vi "Main.vi"() -> ()   [LabVIEW 2011]
uses:
  <vilib>/Utility/miscctls.llb/LVPointTypeDef.ctl
  typedefs/control_references_cluster.ctl
  typedefs/state_cluster.ctl
  typedefs/state_enum.ctl
  <vilib>/DAQmx/write.llb/DAQmx Write (Analog 1D DBL NChan 1Samp).vi
  <vilib>/DAQmx/write.llb/DAQmx Write (Analog 2D DBL NChan NSamp).vi
  subvis/global_image_size.vi
  <vilib>/DAQmx/create/channels.llb/DAQmx Create Channel (AO-Voltage-Basic).vi
  <vilib>/DAQmx/configure/timing.llb/DAQmx Timing (Sample Clock).vi
  <vilib>/DAQmx/miscellaneous.llb/DAQmx Fill In Error Info.vi
  Program Files/National Instruments/LabVIEW 2011/resource/objmgr/daqmx.rc
panel:
  out "SCORE":dbl(knob) scale=0.0..100.0 scale format="%#.0f"
  in  "Play":bool
  in  "Zeit pro Zelle":i32=1 min=1 max=10 step=1
  out "Internal quit":bool
  out "Pfadlänge":dbl format="%#.0f"
  out "Image":picture
  in  "Quit":bool
  out "Signal Qualität":i32(slide) scale=0.0..10.0
  out "Anzahl Neurone":u16(slide) scale=0.0..60.0
  out "Geschwindigkeit":dbl(slide) scale=0.01..1.0 scale format="%#.3g"
  # "Institut für Hirnforschung, UZH"
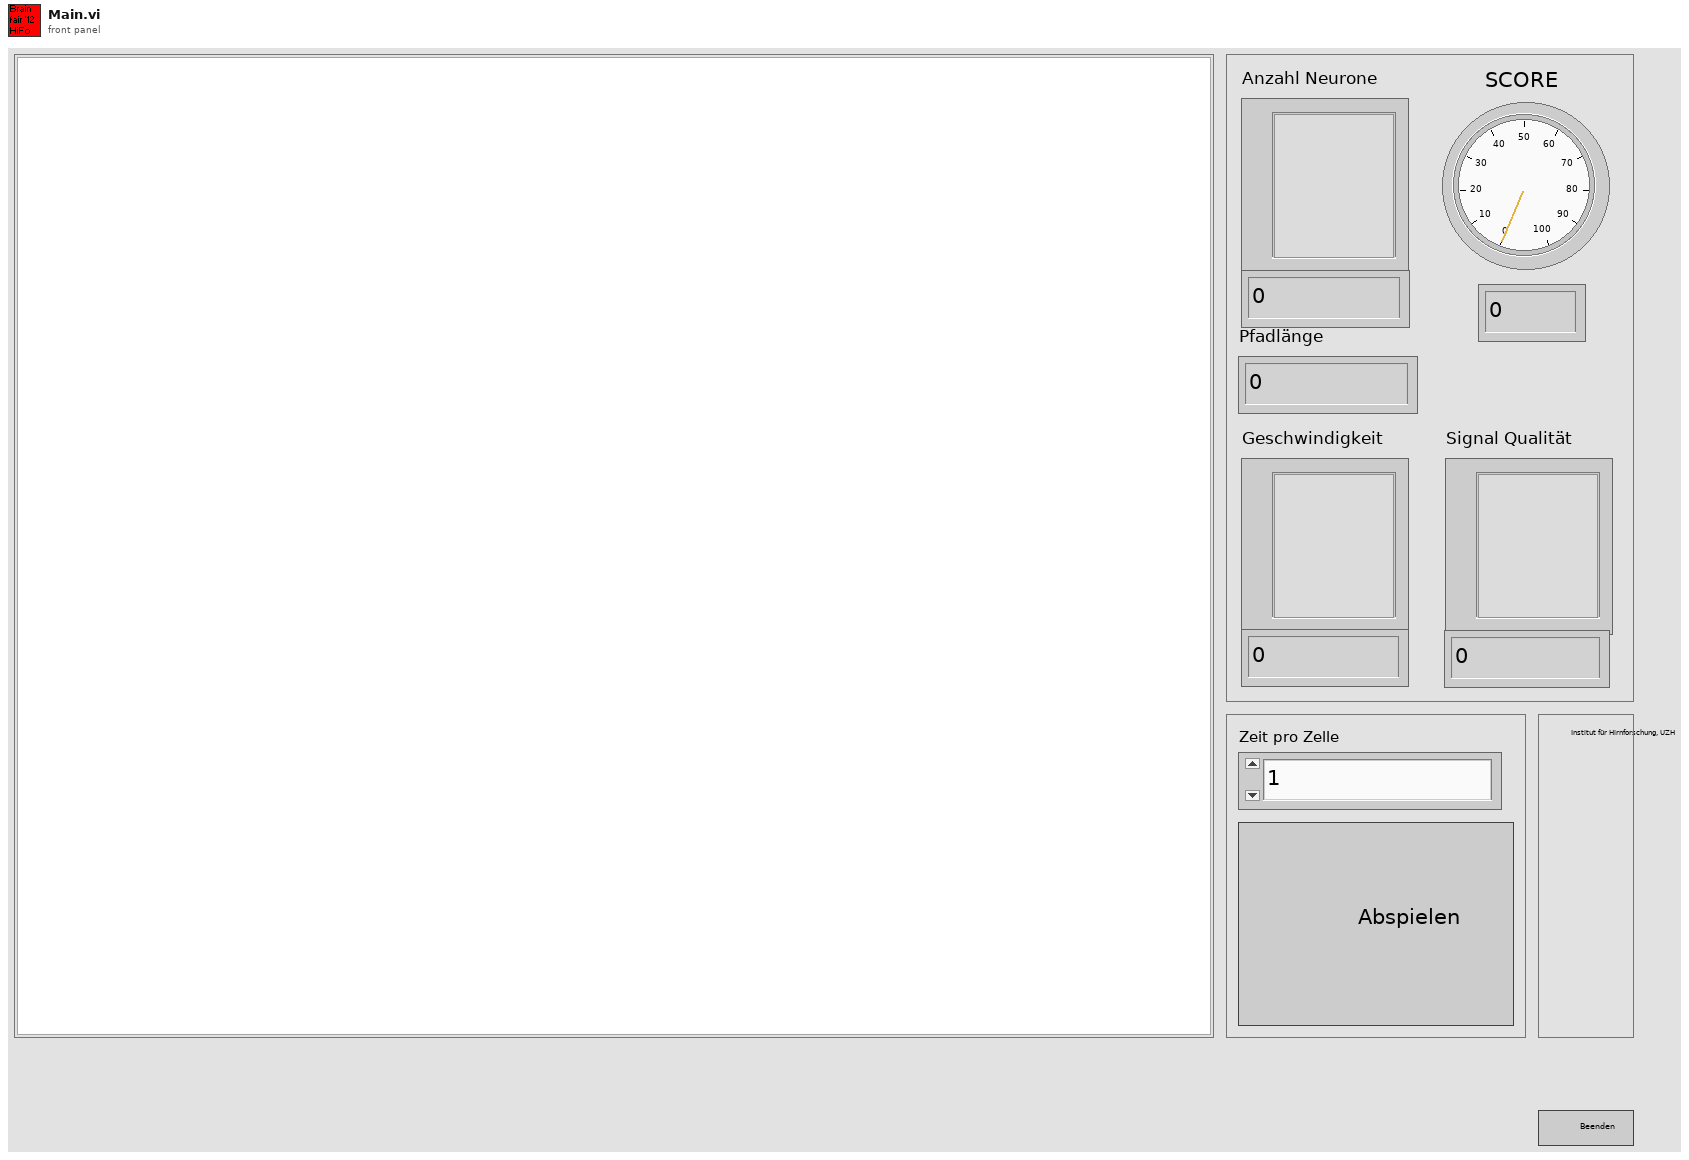
[diagram p1: front panel]
types:
  T1 = typedef "LVPointTypeDef.ctl" = cluster{"Horizontal":i16, "Vertical":i16}
  T2 = typedef "control_references_cluster.ctl" = cluster{"Anzahl Neurone":refnum<vi>, "Zeit pro Zelle":refnum<vi>, "Scan Geschwindigkeit":refnum<vi>, "Pfadlänge":refnum<vi>, "Signal Qualität":refnum<vi>, "SCORE":refnum<vi>}
  T3 = cluster{"Width":u16, "Style":enum32{"Solid", "Dash", "Dot", "DashDot", "DashDotDot"}}
  T4 = typedef "state_cluster.ctl" = cluster{"State":T5, "variant":variant}
  T5 = typedef "state_enum.ctl" = enum16{"Init", "StartSetting", "Moving", "SetNeuron", "FinishSetting", "Quit", "Stop", "Play", "Recalculate"}
  T6 = typedef "LVBoundsTypeDef.ctl" = cluster{"Width":u32, "Height":u32}
  T7 = typedef "LVMouseTypeDef.ctl" = cluster{"Mouse Position":cluster{"X":i32, "Y":i32}, "Mouse Modifiers":cluster{"Button Down":bool, "Shift Mod":bool, "Menu Mod":bool, "Option Mod":bool}}
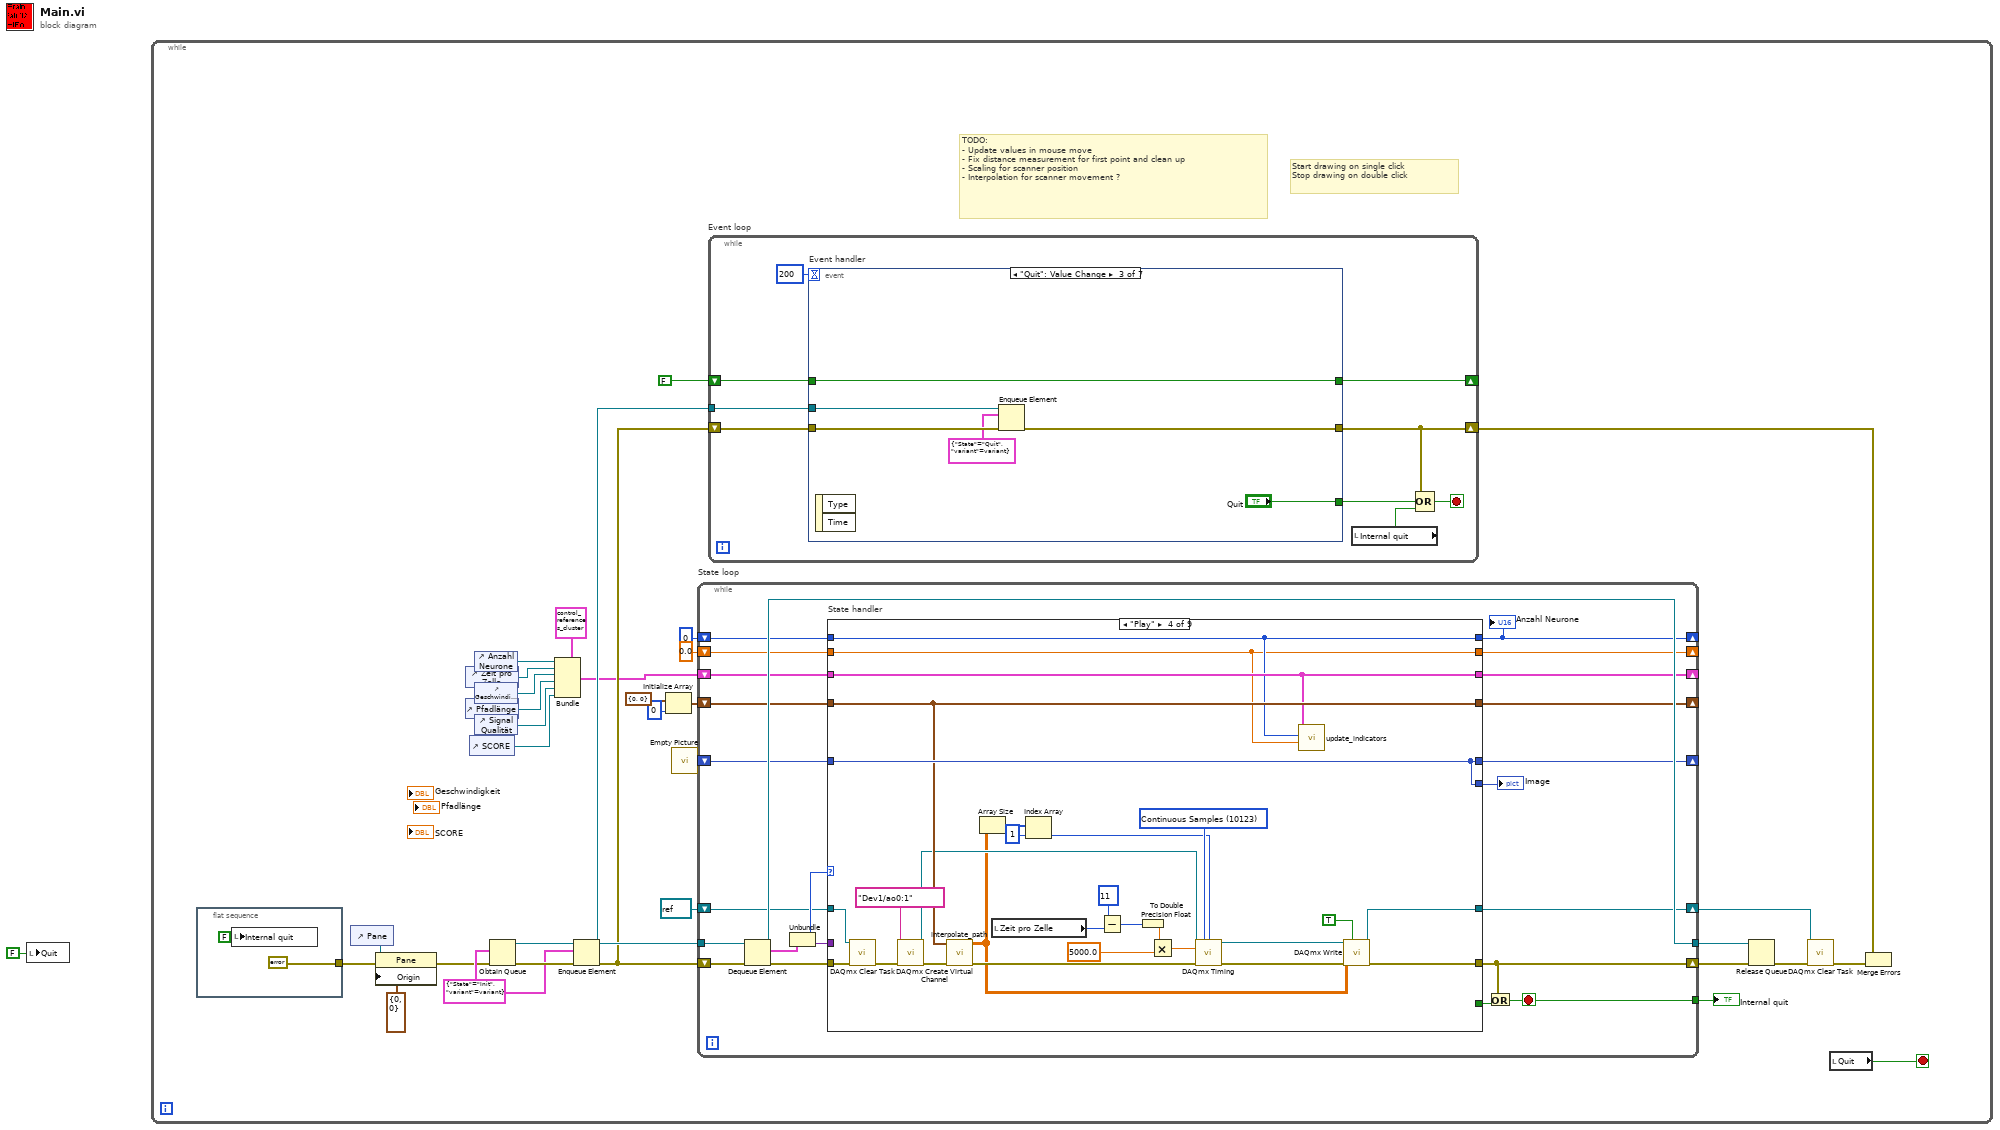
[diagram p0: block diagram]
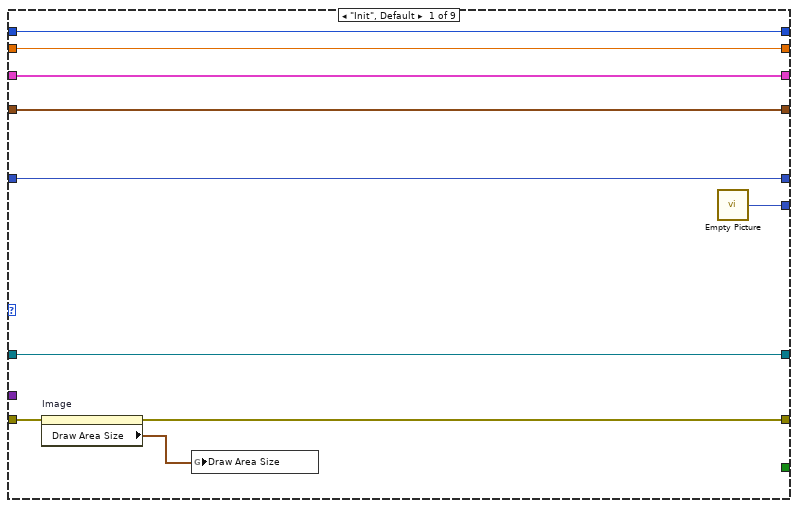
[diagram p2: hidden frame]
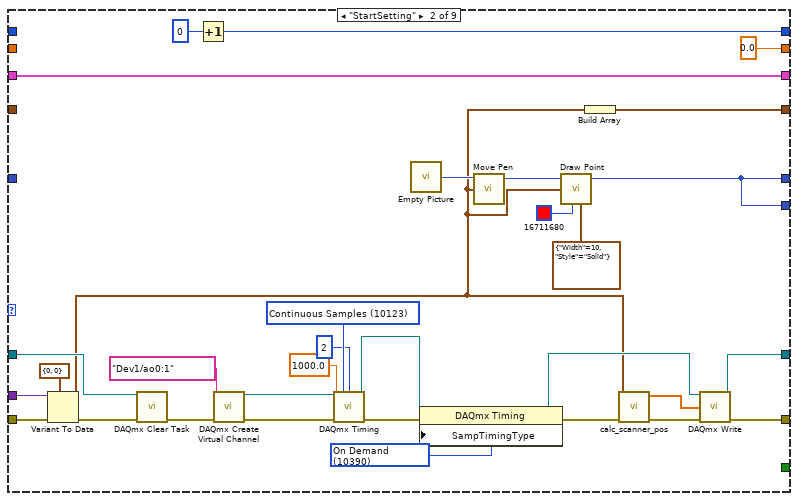
[diagram p3: hidden frame]
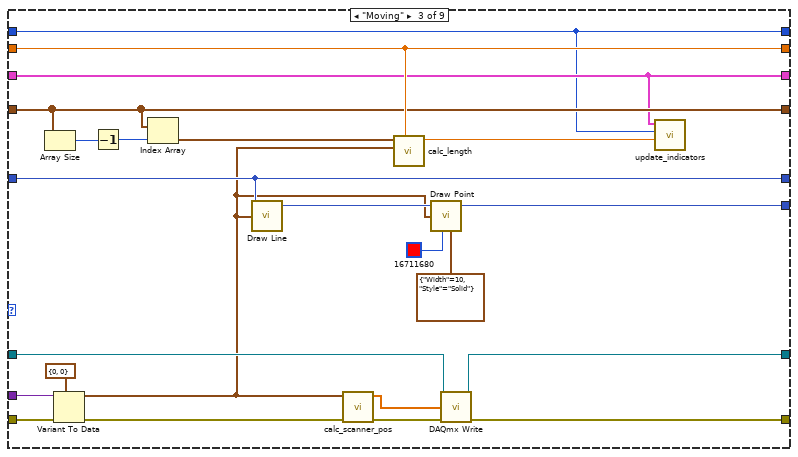
[diagram p4: hidden frame]
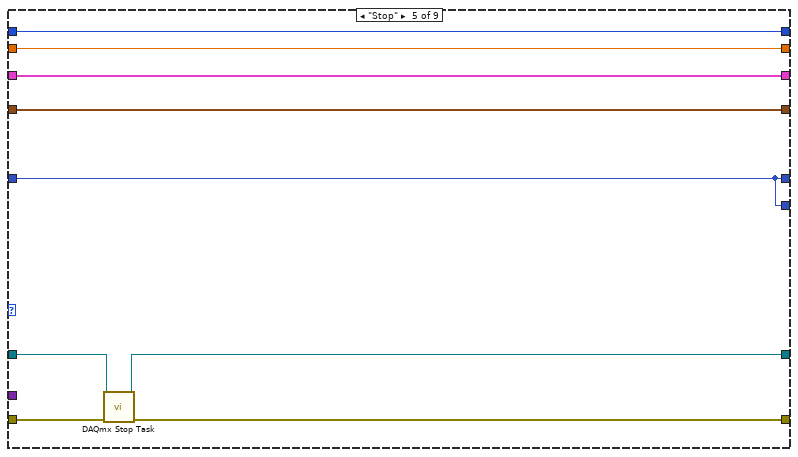
[diagram p5: hidden frame]
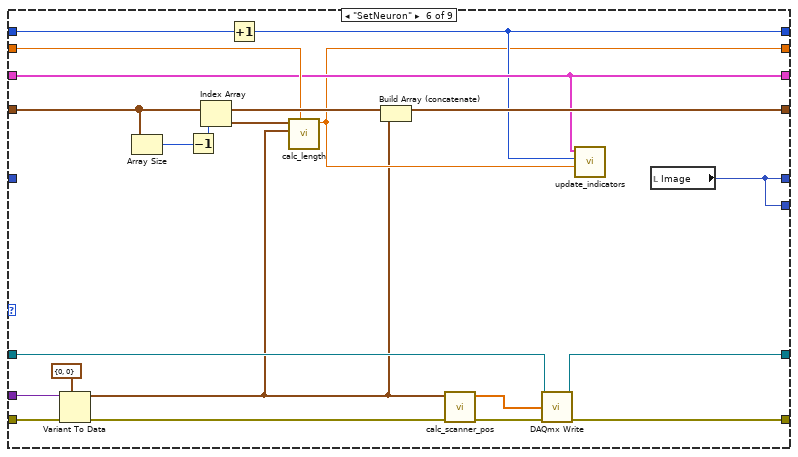
[diagram p6: hidden frame]
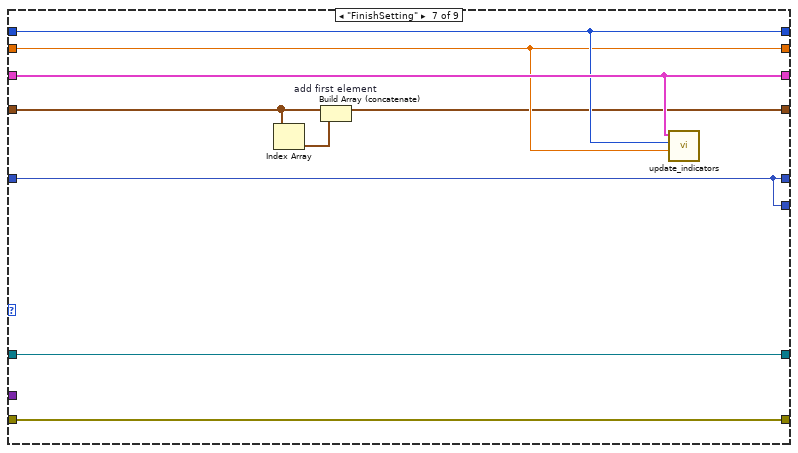
[diagram p7: hidden frame]
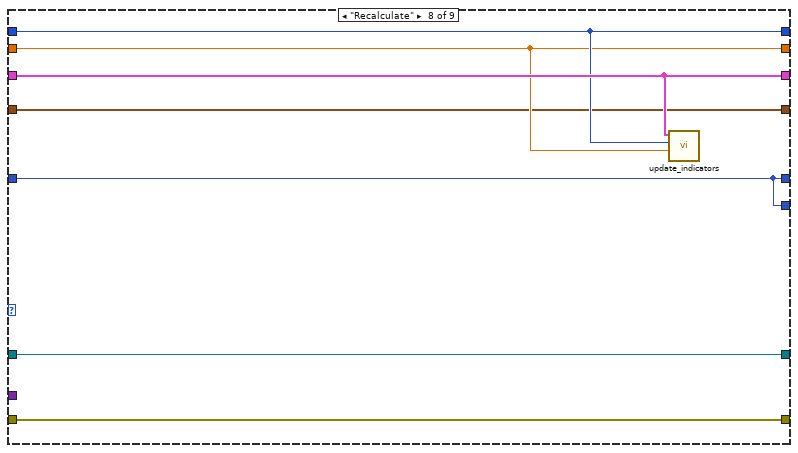
[diagram p8: hidden frame]
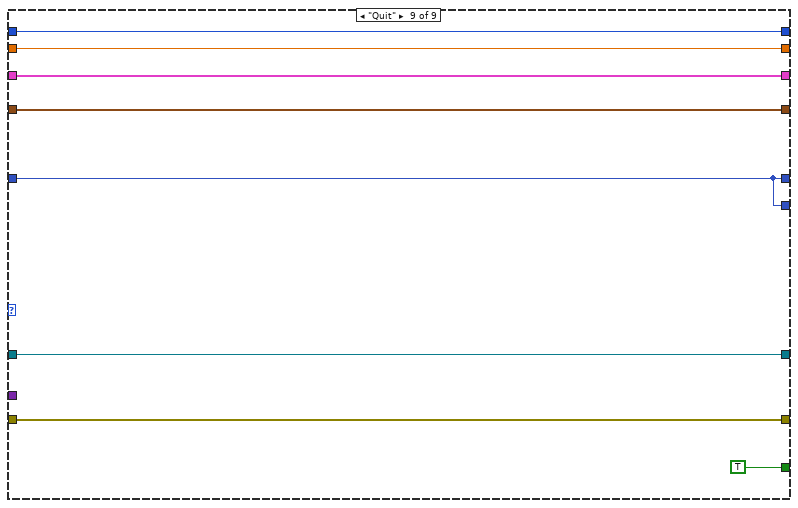
[diagram p9: hidden frame]
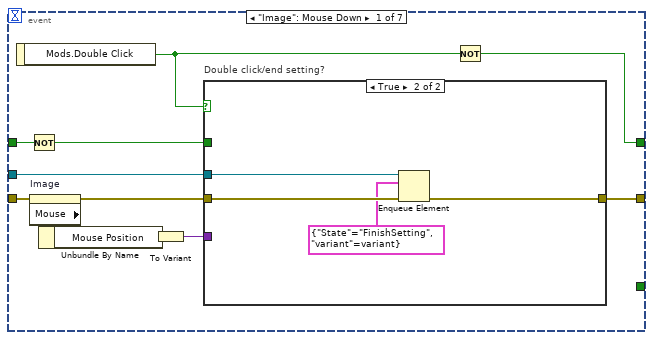
[diagram p10: hidden frame]
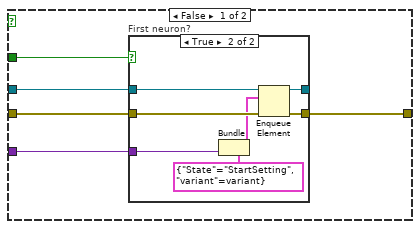
[diagram p11: hidden frame]
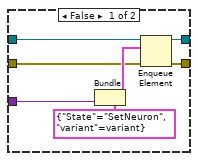
[diagram p12: hidden frame]
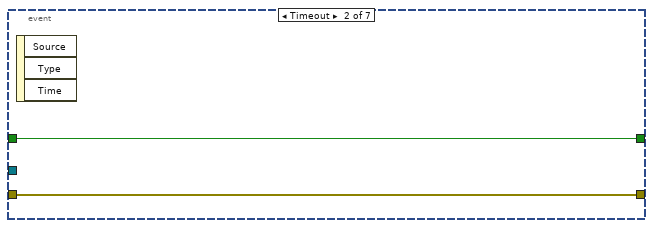
[diagram p13: hidden frame]
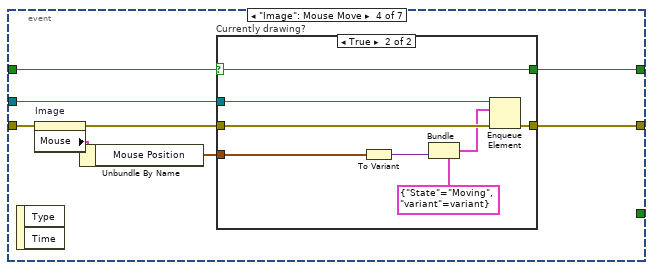
[diagram p14: hidden frame]
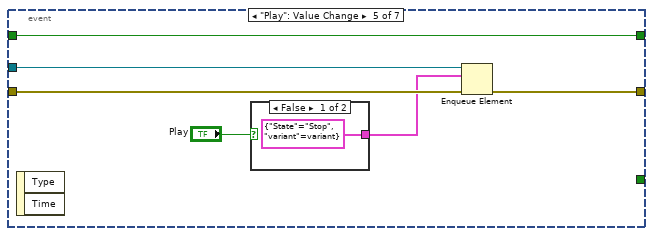
[diagram p16: hidden frame]
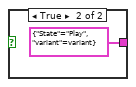
[diagram p17: hidden frame]
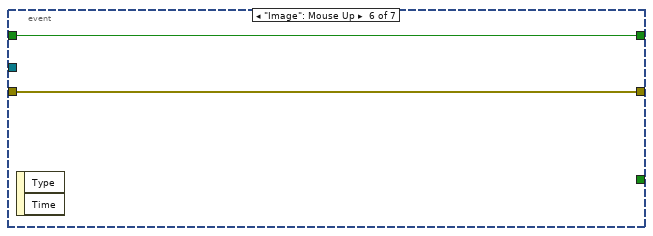
[diagram p18: hidden frame]
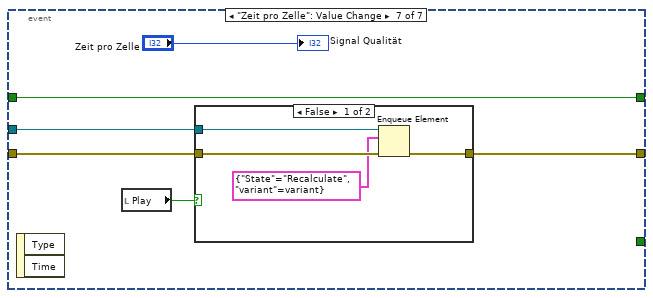
[diagram p19: hidden frame]
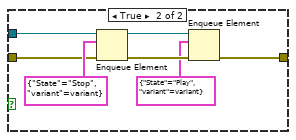
[diagram p20: hidden frame]
diagram:
  n1 = local write "Quit"(FALSE ("Quit")) -> ()
  n2 = while {
    stop <- w3 stop-if-true
    w31 = T4 {"State"=enum."Init", "variant"=variant}
    # "Start drawing on single click\nStop drawing on double click"
    # "TODO:\n- Update values in mouse move\n- Fix distance measurement for first point and clean up\n- Scaling for scanner position\n- Interpolation for scanner movement ?"
    n3 = flat-sequence {
      tunnel: [errorcluster {"status"=FALSE, "code"=0, "source"=""} ("error in (no error)")] -> w5
      frame #0 {
        n4 = local write "Internal quit"(FALSE ("Internal quit")) -> ()
      }
    }
    n5 = control-ref of="Pane"() -> (w7:refnum<vi>)
    n6 = property class="Pane"(reference=w7, error in=w5, "Origin"=T1 {"Horizontal"=0, "Vertical"=0}) -> (error out=w4:errorcluster)  [unwired: 1 out]
    n7 = control-ref of="Zeit pro Zelle"() -> (w13:refnum<vi>)
    n8 = control-ref of="Pfadlänge"() -> (w11:refnum<vi>)
    n9 = control-ref of="SCORE"() -> (w2:refnum<vi>)
    n10 = control-ref of="Anzahl Neurone"() -> (w14:refnum<vi>)
    n11 = control-ref of="Geschwindigkeit"() -> (w12:refnum<vi>)
    n12 = control-ref of="Signal Qualität"() -> (w8:refnum<vi>)
    n13 = Obtain Queue(element data type=w31, error in (no error)=w4) -> (queue out=w32:refnum<queue>, error out=w33:errorcluster)  [unwired: 3 in, 1 out]
    n14 = Bundle(cluster=T2 {"Anzahl Neurone"=refnum, "Zeit pro Zelle"=refnum, "Scan Geschwindigkeit"=refnum, "Pfadlänge"=refnum, "Signal Qualität"=refnum, "SCORE"=refnum} ("output cluster"), "Anzahl Neurone"=w14, "Zeit pro Zelle"=w13, "Scan Geschwindigkeit"=w12, "Pfadlänge"=w11, "Signal Qualität"=w8, "SCORE"=w2) -> (w9:T2)
    n15 = Enqueue Element(queue=w32, element=w31, error in (no error)=w33) -> (queue out=w23:refnum<queue>, error out=w21:errorcluster)  [unwired: 1 in, 1 out]
    n16 = Initialize Array(cluster{"X":i32, "Y":i32} {"X"=0, "Y"=0} ("Mouse Position"), 0 ("dimension size")) -> (w24:cluster{"X":i32, "Y":i32}[])
    n17 = call "Empty Picture"() -> ("empty picture"=w22:picture)
    n18 = while "State loop" {
      shift-right: [w50] -> w30
      shift-left: w21 -> [w57]
      tunnel: w23 -> [w55]
      tunnel: [w51] -> w29
      shift-right: [w39] -> _
      shift-left: u16 0 -> [w48]
      shift-right: [w42] -> _
      shift-left: 0.0 -> [w47]
      shift-right: [w45] -> _
      shift-left: w24 -> [w46]
      shift-right: [w43] -> _
      shift-left: w22 -> [w44]
      tunnel: [w40] -> w20
      shift-right: [w38] -> w15
      shift-left: refnum<k21> refnum ("task out") -> [w37]
      shift-right: [w35] -> _
      shift-left: w9 -> [w36]
      stop <- w40 stop-if-true
      n19 = Dequeue Element(queue=w55, error in (no error)=w57) -> (queue out=w51:refnum<queue>, element=w54:T4, error out=w56:errorcluster)  [unwired: 1 in, 1 out]
      n20 = Unbundle(w54) -> ("State"=w53:T5, "variant"=w52:variant)
      n21 = case "State handler" shown="\"Play\"" w53 {
        tunnel: w56 -> [w62 w98 w121 w135 w155 w179 w189 w196 w198]
        tunnel: [w59 w92 w111 w149 w154 w167 w189 w196 w198] -> w50
        tunnel: w52 -> [_ w97 w120 _ _ w178 _ _ _]
        tunnel: [_ _ _ _ _ _ _ _ TRUE] -> w49
        tunnel: w48 -> [w67 _ w100 w124 w159 w180 w185 w192 w203]
        tunnel: [w67 w94 w100 w124 w159 w162 w185 w192 w203] -> w39
        tunnel: w47 -> [w64 _ w118 w123 w157 w174 w184 w191 w201]
        tunnel: w46 -> [w66 _ w117 w148 w158 w175 w182 w190 w202]
        tunnel: [w66 w68 w117 w148 w158 w176 w181 w190 w202] -> w45
        tunnel: [w64 0.0 w118 w123 w157 w161 w184 w191 w201] -> w42
        tunnel: w44 -> [w65 _ w119 w150 w152 _ w188 w195 w200]
        tunnel: [w65 w88 w119 w150 w152 w173 w188 w195 w200] -> w43
        tunnel: [w63 w88 w106 w150 w152 w173 w188 w195 w200] -> w41
        tunnel: [w58 w91 w109 w147 w151 w165 w187 w194 w199] -> w38
        tunnel: w37 -> [w58 w71 w110 w133 w153 w166 w187 w194 w199]
        tunnel: w36 -> [w60 w84 w101 w125 w156 w163 w186 w193 w197]
        tunnel: [w60 w84 w101 w125 w156 w163 w186 w193 w197] -> w35
        frame "Init", Default {
          n22 = property on="Image" class="Pict"(error in=w62) -> (error out=w59:errorcluster, "Draw Area Size"=w61:T6)  [unwired: 1 in, 1 out]
          n23 = global write "global_image_size.vi" "Draw Area Size"(w61) -> ()
          n24 = call "Empty Picture"() -> ("empty picture"=w63:picture)
        }
        frame "StartSetting" {
          w75 = 10390 items=["Sample Clock"=10388, "Burst Handshake"=12548, "Handshake"=10389, "Implicit"=10451, "On Demand"=10390, "Change Detection"=12504, "Pipelined Sample Clock"=14668] ("SampTimingType")
          w82 = 10123 items=["Finite Samples"=10178, "Continuous Samples"=10123, "Hardware Timed Single Point"=12522] ("sample mode")
          n25 = Variant To Data(error in=w98, type=cluster{"X":i32, "Y":i32} {"X"=0, "Y"=0} ("Mouse Position"), Variant=w97) -> (data=w69:cluster{"X":i32, "Y":i32}, error out=w72:errorcluster)
          n26 = call <vilib>:"DAQmx Clear Task.vi"("task in"=w71, "error in"=w72) -> ("error out"=w70:errorcluster)  [unwired: 13 in]
          n27 = Increment(x=u16 0) -> (x+1=w94:u16)
          n28 = call-poly <vilib>:"DAQmx Create Virtual Channel.vi"("physical channels"=tag "Dev1/ao0:1", "error in"=w70) -> ("task out"=w81:refnum<k21>, "error out"=w83:errorcluster)  [unwired: 12 in]
          n29 = call-poly <vilib>:"DAQmx Timing.vi"("task/channels in"=w81, "sample mode"=w82, "samples per channel"=2, "rate"=1000.0, "error in"=w83) -> ("task out"=w76:refnum<k21>, "error out"=w77:errorcluster)  [unwired: 9 in]
          n30 = call "Empty Picture"() -> ("empty picture"=w96:picture)
          n31 = property class="DAQmx Timing"(reference=w76, error in=w77, "SampTimingType"=w75) -> (reference out=w73:refnum<k21>, error out=w74:errorcluster)
          n32 = call <vilib>:"Move Pen.vi"("new position"=w69, "picture"=w96) -> ("new picture"=w89:picture)  [unwired: 3 in]
          n33 = call <vilib>:"Draw Point.vi"("picture"=w89, "point(x,y)"=w69, "color(black)"=u32 16711680, "pen"=T3 {"Width"=10, "Style"=enum."Solid"}) -> ("new picture"=w88:picture)  [unwired: 5 in]
          n34 = Build Array(w69) -> (w68:cluster{"X":i32, "Y":i32}[])
          n35 = call "calc_scanner_pos.vi"("error in (no error)"=w74, "Mouse position"=w69) -> ("error out"=w93:errorcluster, "Scanner position"=w90:dbl[])  [unwired: 8 in]
          n36 = call-poly <vilib>:"DAQmx Write.vi"("task/channels in"=w73, "data"=w90, "error in"=w93) -> ("task out"=w91:refnum<k21>, "error out"=w92:errorcluster)  [unwired: 10 in, 1 out]
        }
        frame "Moving" {
          n37 = Array Size(array=w117) -> (size(s)=w116:i32)
          n38 = Variant To Data(error in=w121, type=cluster{"X":i32, "Y":i32} {"X"=0, "Y"=0} ("Mouse Position"), Variant=w120) -> (data=w105:cluster{"X":i32, "Y":i32}, error out=w112:errorcluster)
          n39 = Decrement(x=w116) -> (x-1=w115:i32)
          n40 = Index Array(array=w117, index=w115) -> (element=w114:cluster{"X":i32, "Y":i32})
          n41 = call <vilib>:"Draw Line.vi"("picture"=w119, "end point"=w105) -> ("new picture"=w107:picture)  [unwired: 7 in]
          n42 = call "calc_scanner_pos.vi"("error in (no error)"=w112, "Mouse position"=w105) -> ("error out"=w113:errorcluster, "Scanner position"=w108:dbl[])  [unwired: 8 in]
          n43 = call "calc_length.vi"("Old length"=w118, "Current point"=w105, "Last point"=w114) -> ("New length"=w102:dbl)  [unwired: 8 in]
          n44 = call <vilib>:"Draw Point.vi"("picture"=w107, "point(x,y)"=w105, "color(black)"=u32 16711680, "pen"=T3 {"Width"=10, "Style"=enum."Solid"}) -> ("new picture"=w106:picture)  [unwired: 5 in]
          n45 = call-poly <vilib>:"DAQmx Write.vi"("task/channels in"=w110, "data"=w108, "error in"=w113) -> ("task out"=w109:refnum<k21>, "error out"=w111:errorcluster)  [unwired: 10 in, 1 out]
          n46 = call "update_indicators.vi"("New length"=w102, "Neuron number"=w100, "Control references"=w101) -> ()  [unwired: 8 in, 1 out]
        }
        frame "Play" {
          w145 = 10123 items=["Finite Samples"=10178, "Continuous Samples"=10123, "Hardware Timed Single Point"=12522] ("sample mode")
          n47 = call <vilib>:"DAQmx Clear Task.vi"("task in"=w133, "error in"=w135) -> ("error out"=w134:errorcluster)  [unwired: 13 in]
          n48 = call-poly <vilib>:"DAQmx Create Virtual Channel.vi"("physical channels"=tag "Dev1/ao0:1", "error in"=w134) -> ("task out"=w136:refnum<k21>, "error out"=w143:errorcluster)  [unwired: 12 in]
          n49 = call "interpolate_path.vi"("error in (no error)"=w143, "Position Array"=w148) -> ("error out"=w142:errorcluster, "Interploated points"=w132:dbl[][])  [unwired: 8 in]
          n50 = Array Size(array=w132) -> (size(s)=w140:i32[])
          n51 = local read "Zeit pro Zelle"() -> (w127:i32)
          n52 = Index Array(array=w140, index=1) -> (element=w138:i32)
          n53 = Subtract(x=11, y=w127) -> (x-y=w126:i32)
          n54 = To Double Precision Float(number=w126) -> (double precision float=w129:dbl)
          n55 = Multiply(x=w129, y=5000.0 ("rate")) -> (x*y=w130:dbl)
          n56 = call-poly <vilib>:"DAQmx Timing.vi"("task/channels in"=w136, "sample mode"=w145, "samples per channel"=w138, "rate"=w130, "error in"=w142) -> ("task out"=w137:refnum<k21>, "error out"=w141:errorcluster)  [unwired: 9 in]
          n57 = call "update_indicators.vi"("New length"=w123, "Neuron number"=w124, "Control references"=w125) -> ()  [unwired: 8 in, 1 out]
          n58 = call-poly <vilib>:"DAQmx Write.vi"("task/channels in"=w137, "auto start"=TRUE, "data"=w132, "error in"=w141) -> ("task out"=w147:refnum<k21>, "error out"=w149:errorcluster)  [unwired: 9 in, 1 out]
        }
        frame "Stop" {
          n59 = call <vilib>:"DAQmx Stop Task.vi"("task/channels in"=w153, "error in"=w155) -> ("task out"=w151:refnum<k21>, "error out"=w154:errorcluster)  [unwired: 12 in]
        }
        frame "SetNeuron" {
          n60 = Variant To Data(error in=w179, type=cluster{"X":i32, "Y":i32} {"X"=0, "Y"=0} ("Mouse Position"), Variant=w178) -> (data=w160:cluster{"X":i32, "Y":i32}, error out=w168:errorcluster)
          n61 = Array Size(array=w175) -> (size(s)=w171:i32)
          n62 = Decrement(x=w171) -> (x-1=w172:i32)
          n63 = Index Array(array=w175, index=w172) -> (element=w170:cluster{"X":i32, "Y":i32})
          n64 = Increment(x=w180) -> (x+1=w162:u16)
          n65 = call "calc_length.vi"("Old length"=w174, "Current point"=w160, "Last point"=w170) -> ("New length"=w161:dbl)  [unwired: 8 in]
          n66 = Build Array (concatenate)(w175, w160) -> (w176:cluster{"X":i32, "Y":i32}[])
          n67 = call "calc_scanner_pos.vi"("error in (no error)"=w168, "Mouse position"=w160) -> ("error out"=w169:errorcluster, "Scanner position"=w164:dbl[])  [unwired: 8 in]
          n68 = call-poly <vilib>:"DAQmx Write.vi"("task/channels in"=w166, "data"=w164, "error in"=w169) -> ("task out"=w165:refnum<k21>, "error out"=w167:errorcluster)  [unwired: 10 in, 1 out]
          n69 = call "update_indicators.vi"("New length"=w161, "Neuron number"=w162, "Control references"=w163) -> ()  [unwired: 8 in, 1 out]
          n70 = local read "Image"() -> (w173:picture)
        }
        frame "FinishSetting" {
          n71 = Index Array(array=w182) -> (element=w183:cluster{"X":i32, "Y":i32})  [unwired: 1 in]
          n72 = Build Array (concatenate) "add first element"(w182, w183) -> (w181:cluster{"X":i32, "Y":i32}[])
          n73 = call "update_indicators.vi"("New length"=w184, "Neuron number"=w185, "Control references"=w186) -> ()  [unwired: 8 in, 1 out]
        }
        frame "Recalculate" {
          n74 = call "update_indicators.vi"("New length"=w191, "Neuron number"=w192, "Control references"=w193) -> ()  [unwired: 8 in, 1 out]
        }
        frame "Quit" {
        }
      }
      "Image" <- w41
      "Anzahl Neurone" <- w39
      n75 = Or(x=w50, y=w49) -> (x .or. y?=w40:bool)
    }
    "Internal quit" <- w20
    n76 = while "Event loop" {
      shift-right: [w209] -> w19
      shift-left: w21 -> [w213]
      shift-right: [w212] -> _
      shift-left: FALSE -> [w211]
      tunnel: w23 -> [w207]
      stop <- w208 stop-if-true
      n77 = event "Event handler" shown="[2] \"Quit\": Value Change" {
        selector: _ -> [_ _ _ _ _ _ _]
        dyn-events: _ -> [_ _ _ _ _ _ _]
        timeout: 200 -> [_ _ _ _ _ _ _]
        tunnel: w213 -> [w224 w249 w253 w262 w278 w283 w288]
        tunnel: [w214 w249 w252 w263 w277 w283 w286] -> w209
        tunnel: [w222 w248 w254 w256 w279 w282 w289] -> w212
        tunnel: w211 -> [w220 w248 w254 w260 w279 w282 w289]
        tunnel: [_ _ "Quit" _ _ _ _] -> w210
        tunnel: w207 -> [w218 _ w251 w257 w276 _ w287]
        event "Image": Mouse Down {
          n78 = event-data() -> ("Mods.Double Click"=w217:bool)  [unwired: 1 in]
          n79 = Not(x=w220) -> (.not. x?=w216:bool)
          n80 = property on="Image" class="Pict"(error in=w224) -> (error out=w219:errorcluster, "Mouse"=w223:T7)  [unwired: 1 in, 1 out]
          n81 = Unbundle By Name(w223) -> ("Mouse Position"=w221:cluster{"X":i32, "Y":i32})
          n82 = To Variant(anything=w221) -> (Variant=w215:variant)
          n83 = case "Double click/end setting?" shown="True" w217 {
            tunnel: w219 -> [w229 w247]
            tunnel: [w225 w246] -> w214
            tunnel: w218 -> [w228 w245]
            tunnel: w216 -> [w227 _]
            tunnel: w215 -> [w226 _]
            frame False {
              n84 = case "First neuron?" shown="True" w227 {
                tunnel: w229 -> [w234 w243]
                tunnel: [w233 w242] -> w225
                tunnel: w228 -> [w232 w241]
                tunnel: [w231 w240] -> _
                tunnel: w226 -> [w230 w238]
                frame False {
                  n85 = Bundle(cluster=T4 {"State"=enum."SetNeuron", "variant"=variant} ("element"), "variant"=w230) -> (w235:T4)  [unwired: 1 in]
                  n86 = Enqueue Element(queue=w232, element=w235, error in (no error)=w234) -> (queue out=w231:refnum<queue>, error out=w233:errorcluster)  [unwired: 1 in, 1 out]
                }
                frame True {
                  n87 = Bundle(cluster=T4 {"State"=enum."StartSetting", "variant"=variant} ("element"), "variant"=w238) -> (w237:T4)  [unwired: 1 in]
                  n88 = Enqueue Element(queue=w241, element=w237, error in (no error)=w243) -> (queue out=w240:refnum<queue>, error out=w242:errorcluster)  [unwired: 1 in, 1 out]
                }
              }
            }
            frame True {
              n89 = Enqueue Element(queue=w245, element=T4 {"State"=enum."FinishSetting", "variant"=variant}, error in (no error)=w247) -> (error out=w246:errorcluster)  [unwired: 1 in, 2 out]
            }
          }
          n90 = Not(x=w217) -> (.not. x?=w222:bool)
        }
        event Timeout {
          n91 = event-data() -> ()  [unwired: 1 in, 3 out]
        }
        event "Quit": Value Change {
          n92 = event-data() -> ()  [unwired: 1 in, 2 out]
          n93 = Enqueue Element(queue=w251, element=T4 {"State"=enum."Quit", "variant"=variant}, error in (no error)=w253) -> (error out=w252:errorcluster)  [unwired: 1 in, 2 out]
        }
        event "Image": Mouse Move {
          n94 = event-data() -> ()  [unwired: 1 in, 2 out]
          n95 = property on="Image" class="Pict"(error in=w262) -> (error out=w261:errorcluster, "Mouse"=w259:T7)  [unwired: 1 in, 1 out]
          n96 = Unbundle By Name(w259) -> ("Mouse Position"=w258:cluster{"X":i32, "Y":i32})
          n97 = case "Currently drawing?" shown="True" w260 {
            selector: w260 -> [w264 w266]
            tunnel: [w265 w272] -> w263
            tunnel: w261 -> [w265 w273]
            tunnel: w258 -> [_ w268]
            tunnel: w257 -> [_ w271]
            tunnel: [w264 w266] -> w256
            frame False {
            }
            frame True {
              n98 = To Variant(anything=w268) -> (Variant=w269:variant)
              n99 = Bundle(cluster=T4 {"State"=enum."Moving", "variant"=variant} ("element"), "variant"=w269) -> (w267:T4)  [unwired: 1 in]
              n100 = Enqueue Element(queue=w271, element=w267, error in (no error)=w273) -> (error out=w272:errorcluster)  [unwired: 1 in, 2 out]
            }
          }
        }
        event "Play": Value Change {
          n101 = event-data() -> ()  [unwired: 1 in, 2 out]
          n102 = case shown="False" "Play" {
            tunnel: [T4 {"State"=enum."Stop", "variant"=variant} ("element") T4 {"State"=enum."Play", "variant"=variant} ("element")] -> w275
            frame False {
            }
            frame True {
            }
          }
          n103 = Enqueue Element(queue=w276, element=w275, error in (no error)=w278) -> (error out=w277:errorcluster)  [unwired: 1 in, 2 out]
        }
        event "Image": Mouse Up {
          n104 = event-data() -> ()  [unwired: 1 in, 2 out]
        }
        event "Zeit pro Zelle": Value Change {
          n105 = event-data() -> ()  [unwired: 1 in, 2 out]
          n106 = local read "Play"() -> (w285:bool)
          n107 = case shown="False" w285 {
            tunnel: w288 -> [w293 w299]
            tunnel: w287 -> [w291 w298]
            tunnel: [w292 w294] -> w286
            frame False {
              n108 = Enqueue Element(queue=w291, element=T4 {"State"=enum."Recalculate", "variant"=variant}, error in (no error)=w293) -> (error out=w292:errorcluster)  [unwired: 1 in, 2 out]
            }
            frame True {
              n109 = Enqueue Element(queue=w298, element=T4 {"State"=enum."Stop", "variant"=variant}, error in (no error)=w299) -> (queue out=w296:refnum<queue>, error out=w297:errorcluster)  [unwired: 1 in, 1 out]
              n110 = Enqueue Element(queue=w296, element=T4 {"State"=enum."Play", "variant"=variant}, error in (no error)=w297) -> (error out=w294:errorcluster)  [unwired: 1 in, 2 out]
            }
          }
          "Signal Qualität" <- "Zeit pro Zelle"
        }
      }
      n111 = local read "Internal quit"() -> (w206:bool)
      n112 = Compound Arithmetic op=OR(w209, w210, w206) -> (w208:bool)
    }
    n113 = Release Queue(queue=w29, error in (no error)=w30) -> (error out=w17:errorcluster)  [unwired: 1 in, 2 out]
    n114 = call <vilib>:"DAQmx Clear Task.vi"("task in"=w15, "error in"=w17) -> ("error out"=w16:errorcluster)  [unwired: 13 in]
    n115 = local read "Quit"() -> (w3:bool)
    n116 = Merge Errors(w19, w16) -> ()  [unwired: 1 out]
  }
